vi "AttrMap-SetValue2.vi"(8 "error in (no error)":errorcluster, 9 "Value":variant, 10 "Key":string, 11 "AttrMap in":T1) -> (0 "error out":errorcluster, 3 "AttrMap out":T1)   [LabVIEW 2019, in "lv-apt-json-file.lvlib"]
uses:
  Def-AttrMap.ctl
  6e91e2cf-a420-477d-bf86-627245081caf.vi
  lv-apt-json-file.lvlib
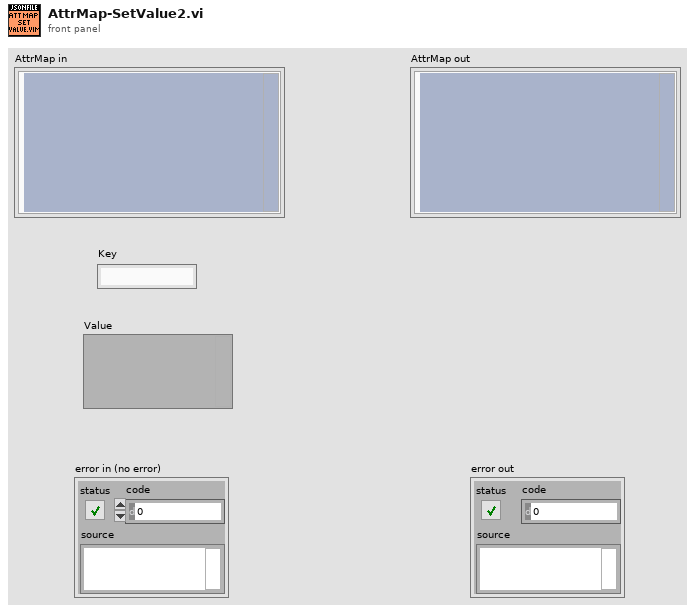
[diagram p1: front panel]
types:
  T1 = typedef "lv-apt-json-file.lvlib/Def-AttrMap.ctl" = cluster{"Map":variant}
  T2 = typedef "lv-apt-json-file.lvlib/Def-AttrMap -- Map.ctl" = map{string, string}
  T3 = typedef "Type Descriptor Enumeration__ogtk.ctl" = enum8{"<Null>", "I8", "I16", "I32", "I64", "U8", "U16", "U32", "U64", "SGL", "DBL", "EXT", "CSG", "CDB", "CXT", "0x0F", "0x10", "0x11", "0x12", "0x13", "0x14", "Enum U8", "Enum U16", "Enum U32", "Enum U64", "SGL PQ", "DBL PQ", "EXT PQ", "CSG PQ", "CDB PQ", "CXT PQ", "0x1F", "0x20", "Boolean", "0x22", "0x23", "0x24", "0x25", "0x26", "0x27", "0x28", "0x29", "0x2A", "0x2B", "0x2C", "0x2D", "0x2E", "0x2F", "String", "0x31", "Path", "Pict", "0x34", "0x35", "0x36", "DAQ", "0x38", "0x39", "0x3A", "0x3B", "0x3C", "0x3D", "0x3E", "0x3F", "Array", "0x41", "0x42", "0x43", "0x44", "0x45", "0x46", "0x47", "0x48", "0x49", "0x4A", "0x4B", "0x4C", "0x4D", "0x4E", "0x4F", "Cluster", "0x51", "0x52", "Variant", "Waveform", "0x55", "0x56", "0x57", "0x58", "0x59", "0x5A", "0x5B", "0x5C", "0x5D", "0x5E", "0x5F", "0x60", "0x61", "0x62", "0x63", "0x64", "0x65", "0x66", "0x67", "0x68", "0x69", "0x6A", "0x6B", "0x6C", "0x6D", "0x6E", "0x6F", "Refnum"}
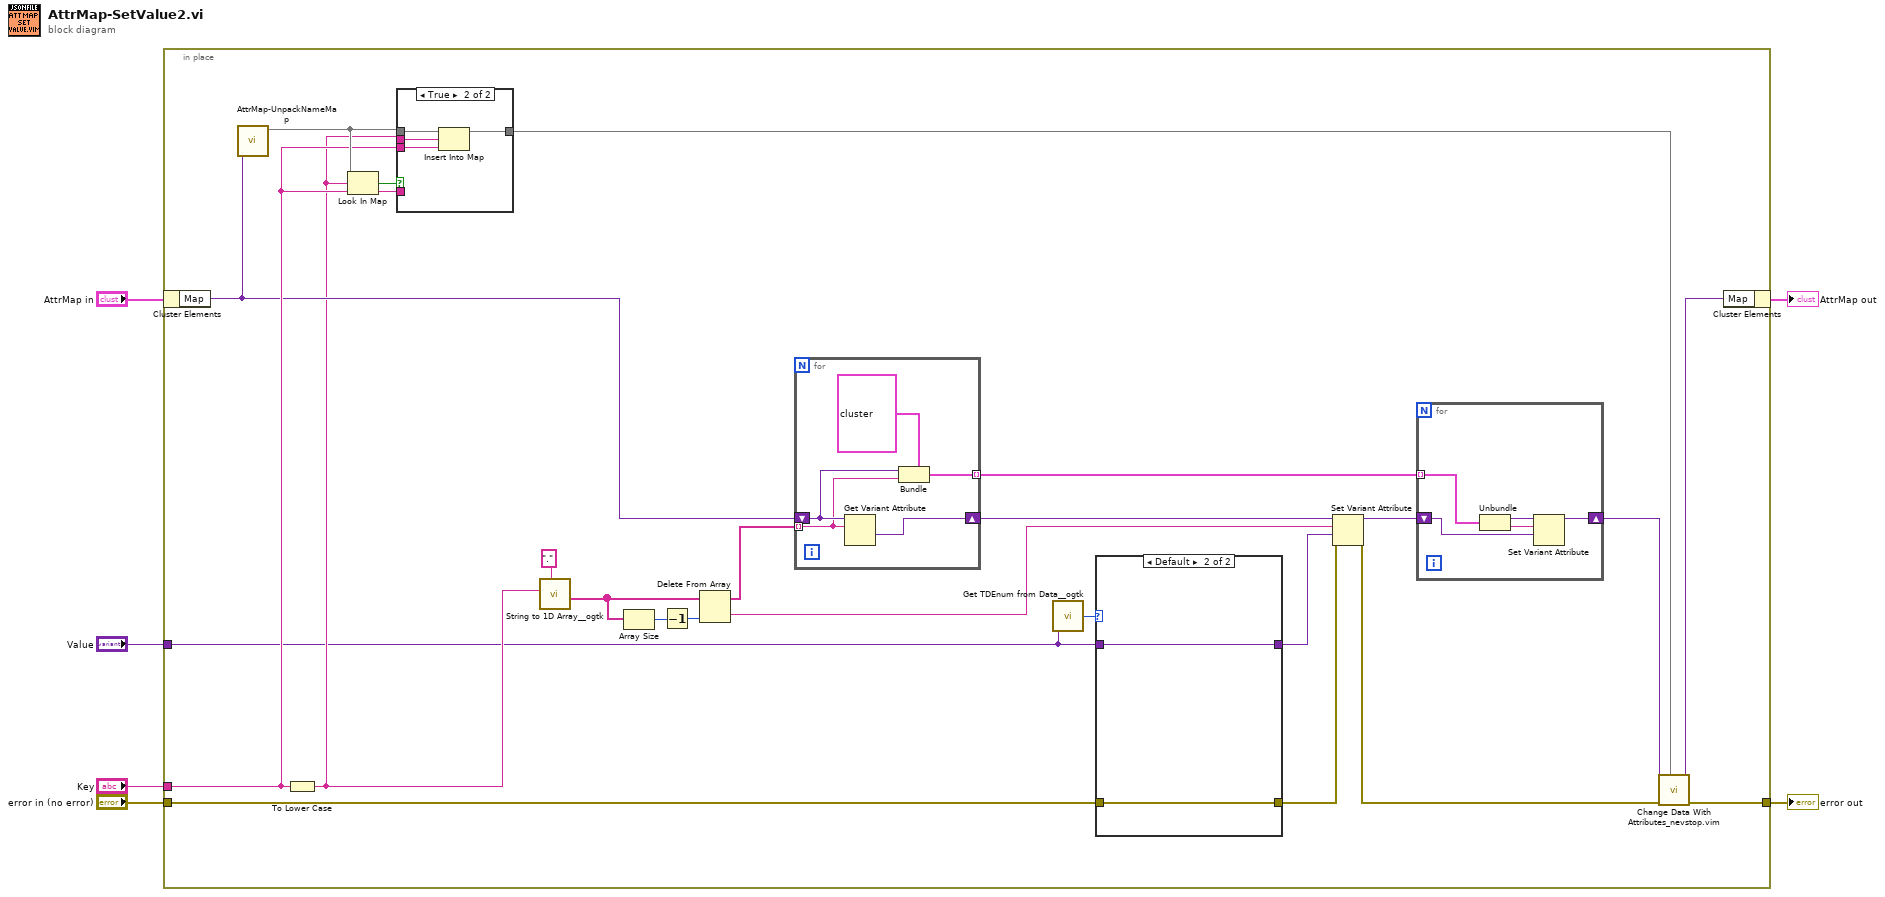
[diagram p0: block diagram]
diagram:
  n1 = in-place {
    in-place-border: [w31] -> w6
    in-place-border: "error in (no error)" -> [w30]
    in-place-border: "Key" -> [w20]
    in-place-border: "Value" -> [w15]
    n2 = in-place-cluster #1("AttrMap in") -> ("Map"=w18:variant)
    n3 = call "AttrMap-UnpackNameMap.vi"("Map"=w18) -> ("NameMap"=w21:T2)  [unwired: 10 in]
    n4 = To Lower Case(string=w20) -> (all lower case string=w16:string)
    n5 = Look In Map(map=w21, key=w16, default value=w20) -> (key not found?=w24:bool, value=w23:string)
    n6 = case shown="True" w24 {
      tunnel: w21 -> [w42 w46]
      tunnel: [w42 w45] -> w25
      tunnel: w16 -> [_ w44]
      tunnel: w20 -> [_ w43]
      tunnel: w23 -> [_ _]
      frame False {
      }
      frame True {
        n7 = Insert Into Map(map in=w46, key=w44, value=w43) -> (map out=w45:T2)  [unwired: 2 out]
      }
    }
    n8 = call <userlib>:"String to 1D Array__ogtk.vi"("delimiter (Tab)"=".", "string"=w16) -> ("Array of Strings"=w12:string[])  [unwired: 9 in]
    n9 = Array Size(array=w12) -> (size(s)=w17:i32)
    n10 = Decrement(x=w17) -> (x-1=w7:i32)
    n11 = Delete From Array(array=w12, index=w7) -> (deleted portion=w13:string, array with subset deleted=w11:string[])  [unwired: 1 in]
    n12 = for {
      tunnel: w11 -> [w40] mode=indexing
      shift-right: [w39] -> w14
      shift-left: w18 -> [w41]
      tunnel: [w37] -> w10 mode=indexing
      n13 = Get Variant Attribute(Variant=w41, name=w40) -> (value=w39:variant)  [unwired: 2 in, 3 out]
      n14 = Bundle(cluster=cluster{"Parent":variant, "Name":string} {"Parent"=variant, "Name"=""}, "Parent"=w41, "Name"=w40) -> (w37:cluster{"Parent":variant, "Name":string})
    }
    n15 = call <userlib>:"Get TDEnum from Data__ogtk.vi"("Data"=w15) -> ("Type Descriptor Enumeration"=w27:T3)  [unwired: 4 in]
    n16 = case shown="Default" w27 {
      tunnel: w15 -> [w48 w49]
      tunnel: w30 -> [w47 w50]
      tunnel: [w47 w50] -> w29
      tunnel: [w48 w49] -> w28
      frame "Cluster" {
      }
      frame Default {
      }
    }
    n17 = Set Variant Attribute(Variant=w14, name=w13, value=w28, error in=w29) -> (Variant out=w9:variant, error out=w26:errorcluster)  [unwired: 1 out]
    n18 = for {
      tunnel: w10 -> [w36] mode=indexing
      shift-right: [w35] -> w8
      shift-left: w9 -> [w32]
      n19 = Unbundle(w36) -> ("Parent"=w34:variant, "Name"=w33:string)
      n20 = Set Variant Attribute(Variant=w34, name=w33, value=w32) -> (Variant out=w35:variant)  [unwired: 1 in, 2 out]
    }
    n21 = call "Change Data With Attributes_nevstop.vim"("Data"=w25, "error in (no error)"=w26, "Variant in"=w8) -> ("error out"=w31:errorcluster, "Variant out"=w22:variant)  [unwired: 7 in]
    n22 = in-place-cluster #1("Map"=w22) -> (→"AttrMap out":T1)
  }
  "error out" <- w6
